vi "MGCC_EnergyMgmt_main.vi"   [LabVIEW 2016]
doc: "-----------------------------------------------------------------------------------------------------------------------\nCopyright <2019> <The University of Tennessee at Knoxville and the University of Tennessee Research Foundation>\nThis software is released under BSD-3 \nhttps://opensource.org/licenses/BSD-3-Clause \nAdditional license options available at https://utrf.tennessee.edu/industry/sample-agreements/\n-----------------------------------------------------------------------------------------------------------------------\n\nThis VI implements the Energy Management function in the MGCC. Linear programming is used to minimize electricity tariffs in grid-connected mode, and plan for islanded operation for the next 24 hours (can be changed) in islanded mdoe. The VI calls \"MGCC_EnergyMgmt_EMS_HTB.vi\" every hour."
uses:
  Finite State Machine/Sub-VIs/MGCC_FntStaMach_gobal.vi
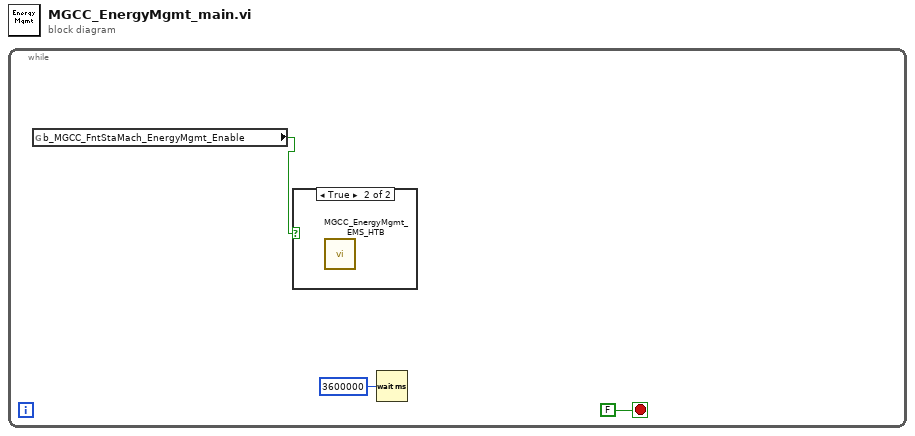
[diagram p0: block diagram]
diagram:
  n1 = while {
    stop <- FALSE stop-if-true
    n2 = global read "MGCC_FntStaMach_gobal.vi" "b_MGCC_FntStaMach_EnergyMgmt_Enable"() -> (w1:bool)
    n3 = case shown="True" w1 {
      frame False {
      }
      frame True {
        n4 = call "MGCC_EnergyMgmt_EMS_HTB.vi"() -> ()  [unwired: 12 in]
      }
    }
    n5 = Wait (ms)(milliseconds to wait=u32 3600000) -> ()  [unwired: 1 out]
  }
